vi "Advance past Object.vi"(7 "JSON":string, 9 "Offset":i32) -> (1 "Offset past Object":i32, 2 "Object Start":i32, 3 "State":T1)   [LabVIEW 2013, in "JSONtext.lvlib"]
uses:
  JSONtext.lvlib
  Parsing State.ctl
  Advance past Number.vi
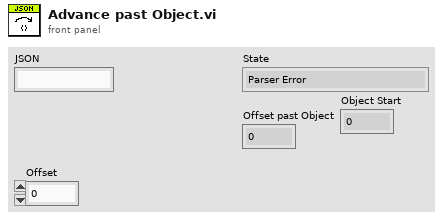
[diagram p1: front panel]
types:
  T1 = typedef "JSONtext.lvlib/Parsing State.ctl" = enum16{"Parser Error", "Object", "Array", "String", "Number/Other", "Leading Whitespace", "Object end", "Array end", "Value end"}
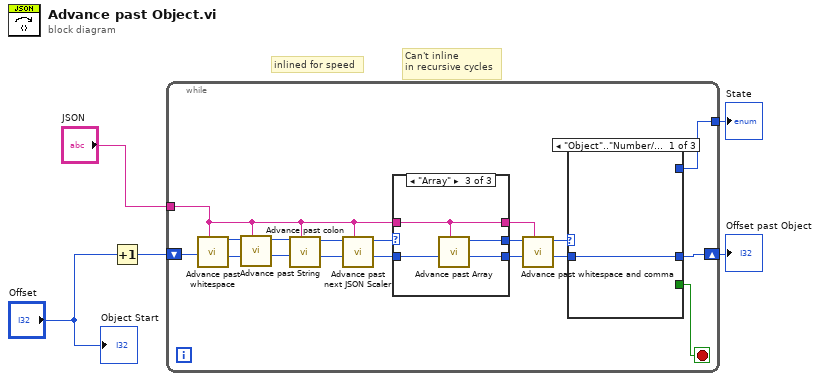
[diagram p0: block diagram]
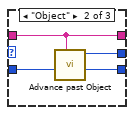
[diagram p3: hidden frame]
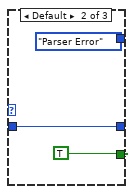
[diagram p4: hidden frame]
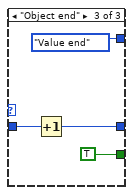
[diagram p5: hidden frame]
diagram:
  # "Can't inline\nin recursive cycles"
  # "inlined for speed"
  n1 = Increment(x="Offset") -> (x+1=w2:i32)
  n2 = while {
    shift-right: [w19] -> w3
    shift-left: w2 -> [w16]
    tunnel: "JSON" -> [w6]
    tunnel: [w17] -> w5
    stop <- w18 stop-if-true
    n3 = call "Advance past whitespace.vi"("JSON"=w6, "Offset"=w16) -> ("Offset of first non-whitespace"=w15:i32, "State"=w14:T1)  [unwired: 8 in]
    n4 = call "Advance past String.vi"("JSON"=w6, "Offset"=w15, "State in"=w14) -> ("Offset past match"=w23:i32, "State"=w22:T1)  [unwired: 6 in, 1 out]
    n5 = call "Advance past colon.vi"("JSON"=w6, "Offset"=w23, "State"=w22) -> ("index"=w8:i32, "State"=w9:T1)  [unwired: 7 in]
    n6 = call "Advance past next JSON Scaler.vi"("JSON"=w6, "Offset"=w8, "State"=w9) -> ("index"=w7:i32, "Enum"=w10:T1)  [unwired: 6 in, 1 out]
    n7 = case shown="\"Array\"" w10 {
      selector: w10 -> [w25 _ _]
      tunnel: w7 -> [w24 w30 w34]
      tunnel: [w25 w29 w33] -> w12
      tunnel: [w24 w28 w32] -> w11
      tunnel: w6 -> [w26 w27 w31]
      tunnel: [w26 w27 w31] -> w13
      frame Default {
      }
      frame "Object" {
        n8 = call "Advance past Object.vi"("JSON"=w27, "Offset"=w30) -> ("Offset past Object"=w28:i32, "State"=w29:T1)  [unwired: 7 in, 1 out]
      }
      frame "Array" {
        n9 = call "Advance past Array.vi"("JSON"=w31, "Offset"=w34) -> ("Offset past match"=w32:i32, "State"=w33:T1)  [unwired: 7 in, 1 out]
      }
    }
    n10 = call "Advance past whitespace and comma.vi"("JSON"=w13, "Offset"=w11, "State in"=w12) -> ("Offset past match"=w21:i32, "State"=w20:T1)  [unwired: 7 in]
    n11 = case shown="\"Object\"..\"Number/Other\"" w20 {
      tunnel: [_ TRUE TRUE] -> w18
      tunnel: [_ Parsing_State."Parser Error" Parsing_State."Value end"] -> w17
      tunnel: w21 -> [w35 w36 w40]
      tunnel: [w35 w36 w39] -> w19
      frame "Object".."Number/Other" {
      }
      frame Default {
      }
      frame "Object end" {
        n12 = Increment(x=w40) -> (x+1=w39:i32)
      }
    }
  }
  "State" <- w5
  "Offset past Object" <- w3
  "Object Start" <- "Offset"
